vi "Write Failure Action.vi"(10 "Failure Action":string, 11 "Change Failure Action in":refnum<class "Change Failure Action.lvclass">) -> (3 "Change Failure Action out":refnum<class "Change Failure Action.lvclass">)   [LabVIEW 2016, in "Assert API Components.lvlib" / "Assert Display.lvlib" / "Main Display.lvlib" / "Change Failure Action.lvclass"]
uses:
  Change Failure Action.lvclass
  Change Failure Action.lvclass/Change Failure Action.ctl
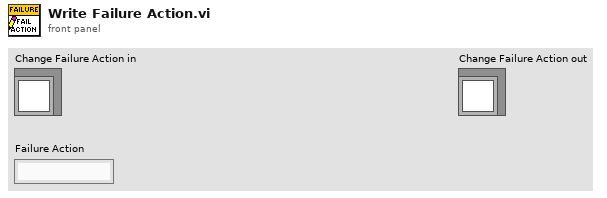
[diagram p1: front panel]
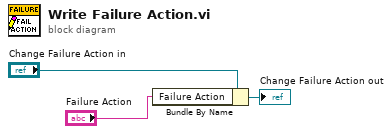
[diagram p0: block diagram]
diagram:
  n1 = Bundle By Name(cluster="Change Failure Action in", "Failure Action"="Failure Action") -> (→"Change Failure Action out":refnum<class "Change Failure Action.lvclass">)
